vi "Get Channels and Messages.vi"(8 "error in":errorcluster, 11 "custom device ref":T2 format="%.0x") -> (0 "error out":errorcluster, 1 "outgoing channels":T2[](array[typedef]) format="%.0x", 2 "incoming channels":T2[](array[typedef]) format="%.0x", 3 "custom device ref out":T2 format="%.0x", 4 "transmitted messages":T1[](array[typedef]) {"Message Section Handle" format="%.0x"; "Parameter Channel Handles" format="%.0x"}, 6 "received messages":T1[](array[typedef]) {"Message Section Handle" format="%.0x"; "Parameter Channel Handles" format="%.0x"})   [LabVIEW 2020, in "AIM MIL-STD-1553 Engine.lvlib" / "Implementation.lvlib" / "Execution Unit.lvclass"]
uses:
  Execution Unit.lvclass
  <vilib>/NI VeriStand/Custom Device API/Custom Device Item Ref.ctl
  Custom Device/Compiled Message.ctl
  Shared/Direction.ctl
  Shared/Parameter Definition.ctl
  <vilib>/NI VeriStand/Custom Device API/Custom Device API.lvlib
  Scripting/AIM MIL-STD-1553 Scripting.lvlib
  Custom Device/Custom Device.lvlib
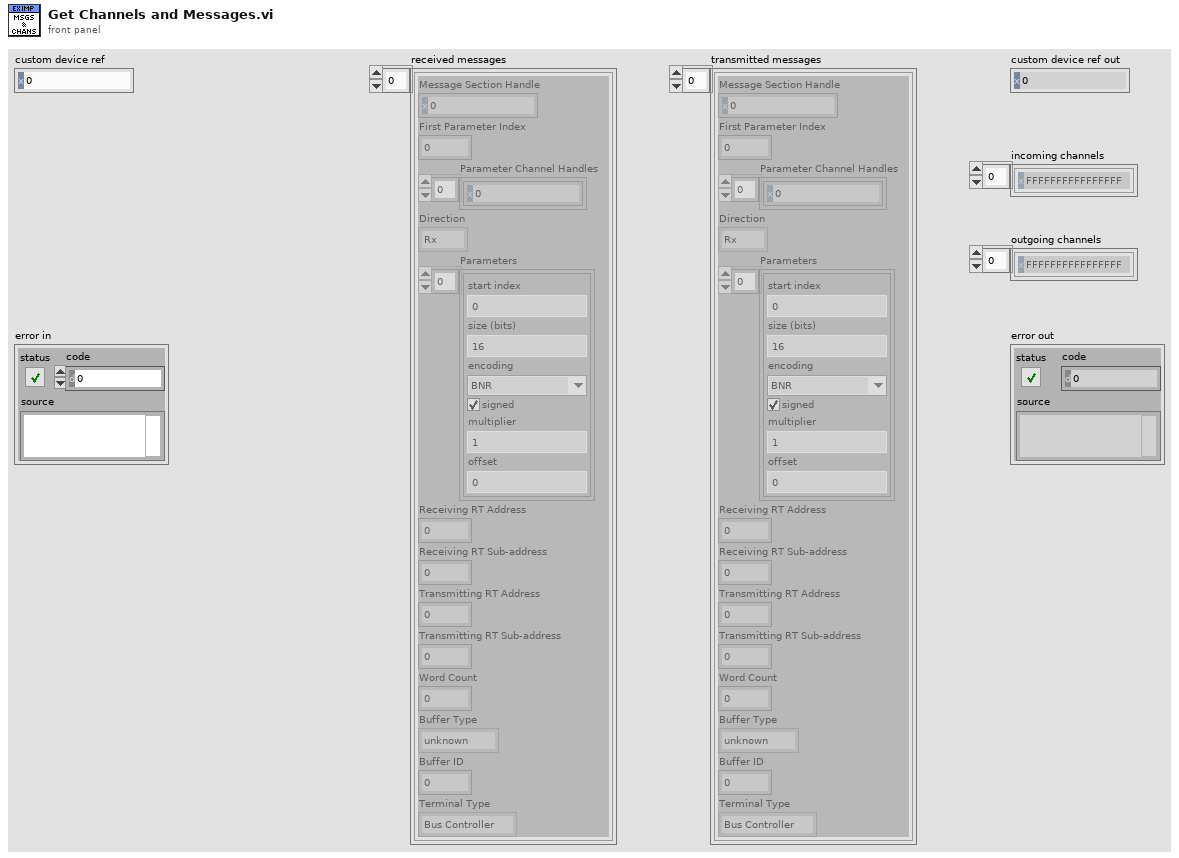
[diagram p1: front panel]
types:
  T1 = typedef "AIM MIL-STD-1553 Engine.lvlib/Custom Device.lvlib/Compiled Message.ctl" = cluster{"Message Section Handle":T2, "First Parameter Index":i32, "Parameter Channel Handles":T2[], "Direction":T3, "Parameters":T4[], "Receiving RT Address":u8, "Receiving RT Sub-address":u8, "Transmitting RT Address":u8, "Transmitting RT Sub-address":u8, "Word Count":u8, "Buffer Type":enum16{"unknown", "BC Message Buffer", "RT Message Buffer"}, "Buffer ID":u16, "Terminal Type":enum16{"Bus Controller", "Remote Terminal"}}
  T2 = typedef "Custom Device API.lvlib/Custom Device Item Ref.ctl" = u64
  T3 = typedef "Direction.ctl" = enum16{"Rx", "Tx"}
  T4 = typedef "Parameter Definition.ctl" = cluster{"start index":i32, "size (bits)":i32, "encoding":enum16{"BNR", "BCD", "Discrete"}, "signed":bool, "multiplier":dbl, "offset":dbl}
  T5 = typedef "Terminal Endpoint.ctl" = cluster{"terminal address":T6, "subaddress":T6}
  T6 = typedef "Address.ctl" = u16
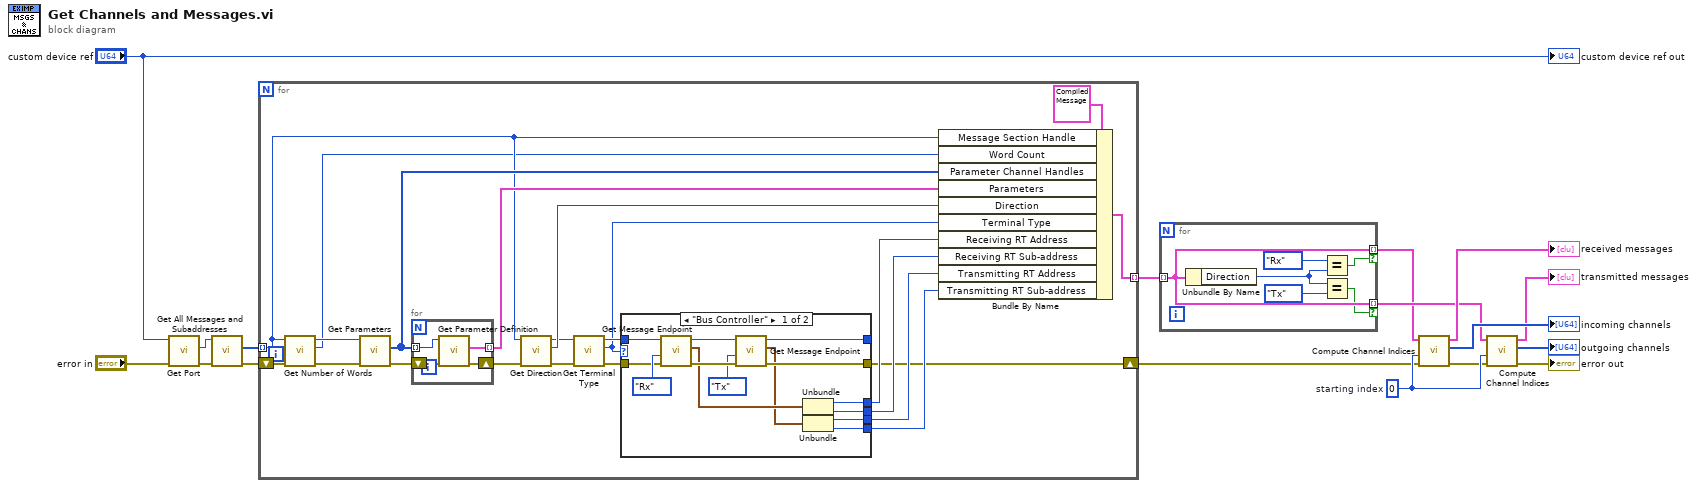
[diagram p0: block diagram]
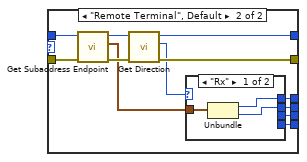
[diagram p2: hidden frame]
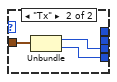
[diagram p3: hidden frame]
diagram:
  w12 = 0  # starting index
  n1 = call "Get Port.vi"("error in"="error in", "custom device ref"="custom device ref") -> ("error out"=w4:errorcluster, "port"=w3:T2)  [unwired: 6 in, 2 out]
  n2 = call "Get All Messages and Subaddresses.vi"("error in"=w4, "port"=w3) -> ("error out"=w11:errorcluster, "messages and subaddresses"=w10:T2[])  [unwired: 7 in, 1 out]
  n3 = for {
    shift-right: [w24] -> w6
    shift-left: w11 -> [w22]
    tunnel: w10 -> [w23] mode=indexing
    tunnel: [w39] -> w9 mode=indexing
    n4 = call "Get Number of Words.vi"("error in"=w22, "message or subaddress"=w23) -> ("error out"=w21:errorcluster, "number of words"=w19:u16, "message or subaddress out"=w20:T2)  [unwired: 7 in]
    n5 = call "Get Parameters.vi"("error in"=w21, "message or subaddress"=w20) -> ("error out"=w36:errorcluster, "parameters"=w35:T2[])  [unwired: 7 in, 1 out]
    n6 = for {
      shift-right: [w75] -> w33
      shift-left: w36 -> [w74]
      tunnel: w35 -> [w73] mode=indexing
      tunnel: [w72] -> w34 mode=indexing
      n7 = call "Get Parameter Definition.vi"("error in"=w74, "parameter"=w73) -> ("error out"=w75:errorcluster, "parameter definition"=w72:T4)  [unwired: 7 in, 1 out]
    }
    n8 = call "Get Direction.vi"("error in"=w33, "message or subaddress"=w23) -> ("error out"=w30:errorcluster, "direction"=w37:T3, "message or subaddress out"=w29:T2)  [unwired: 6 in, 1 out]
    n9 = call "Get Terminal Type.vi"("error in"=w30, "message or subaddress"=w29) -> ("error out"=w32:errorcluster, "terminal type"=w18:enum16{"Bus Controller", "Remote Terminal"}, "message or subaddress out"=w31:T2)  [unwired: 7 in]
    n10 = case shown="\"Bus Controller\"" w18 {
      tunnel: [w47 w63] -> _
      tunnel: [w46 w62] -> w24
      tunnel: w31 -> [w53 w59]
      tunnel: w32 -> [w51 w58]
      tunnel: [w40 w57] -> w25
      tunnel: [w41 w56] -> w26
      tunnel: [w44 w55] -> w27
      tunnel: [w45 w54] -> w28
      frame "Bus Controller" {
        n11 = call "Get Message Endpoint.vi"("error in"=w51, "direction"=Direction."Rx", "message"=w53) -> ("error out"=w50:errorcluster, "remote terminal endpoint"=w43:T5, "message out"=w48:T2)  [unwired: 5 in, 1 out]
        n12 = call "Get Message Endpoint.vi"("error in"=w50, "direction"=Direction."Tx", "message"=w48) -> ("error out"=w46:errorcluster, "remote terminal endpoint"=w42:T5, "message out"=w47:T2)  [unwired: 5 in, 1 out]
        n13 = Unbundle(w43) -> ("terminal address"=w45:T6, "subaddress"=w44:T6)
        n14 = Unbundle(w42) -> ("terminal address"=w41:T6, "subaddress"=w40:T6)
      }
      frame "Remote Terminal", Default {
        n15 = call "Get Subaddress Endpoint.vi"("error in"=w58, "subaddress"=w59) -> ("error out"=w64:errorcluster, "remote terminal endpoint"=w60:T5, "subaddress out"=w65:T2)  [unwired: 7 in]
        n16 = call "Get Direction.vi"("error in"=w64, "message or subaddress"=w65) -> ("error out"=w62:errorcluster, "direction"=w61:T3, "message or subaddress out"=w63:T2)  [unwired: 6 in, 1 out]
        n17 = case shown="\"Rx\"" w61 {
          tunnel: w60 -> [w68 w71]
          tunnel: [w67 _] -> w54
          tunnel: [w66 _] -> w55
          tunnel: [_ w70] -> w56
          tunnel: [_ w69] -> w57
          frame "Rx" {
            n18 = Unbundle(w68) -> ("terminal address"=w67:T6, "subaddress"=w66:T6)
          }
          frame "Tx" {
            n19 = Unbundle(w71) -> ("terminal address"=w70:T6, "subaddress"=w69:T6)
          }
        }
      }
    }
    n20 = Bundle By Name(cluster=T1 {"Message Section Handle"=18446744073709551615, "First Parameter Index"=0, "Parameter Channel Handles"=[], "Direction"=enum."Rx", "Parameters"=[], "Receiving RT Address"=0, "Receiving RT Sub-address"=0, "Transmitting RT Address"=0, "Transmitting RT Sub-address"=0, "Word Count"=0, "Buffer Type"=enum."unknown", "Buffer ID"=0, "Terminal Type"=enum."Bus Controller"}, "Message Section Handle"=w23, "Word Count"=w19, "Parameter Channel Handles"=w35, "Parameters"=w34, "Direction"=w37, "Terminal Type"=w18, "Receiving RT Address"=w28, "Receiving RT Sub-address"=w27, "Transmitting RT Address"=w26, "Transmitting RT Sub-address"=w25) -> (w39:T1)
  }
  n21 = for {
    tunnel: w9 -> [w81] mode=indexing
    tunnel: [w81] -> w7 mode=indexing if=w77
    tunnel: [w81] -> w8 mode=indexing if=w76
    n22 = Unbundle By Name(w81) -> ("Direction"=w80:T3)
    n23 = Equal?(x=Direction."Rx", y=w80) -> (x = y?=w77:bool)
    n24 = Equal?(x=w80, y=Direction."Tx" ("x")) -> (x = y?=w76:bool)
  }
  n25 = call "Compute Channel Indices.vi"("error in (no error)"=w6, "Next Index in"=w12, "Messages in"=w7) -> ("error out"=w5:errorcluster, "Channel Handles"=→"incoming channels":T2[], "Messages out"=→"received messages":T1[])  [unwired: 5 in, 1 out]
  n26 = call "Compute Channel Indices.vi"("error in (no error)"=w5, "Next Index in"=w12, "Messages in"=w8) -> ("error out"=→"error out":errorcluster, "Channel Handles"=→"outgoing channels":T2[], "Messages out"=→"transmitted messages":T1[])  [unwired: 5 in, 1 out]
  "custom device ref out" <- "custom device ref"
